vi "mean.vi"(11 "Array":i16[][](array[numeric])) -> (3 "mean":dbl)   [LabVIEW 2015]
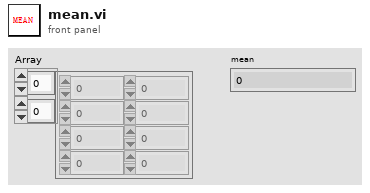
[diagram p1: front panel]
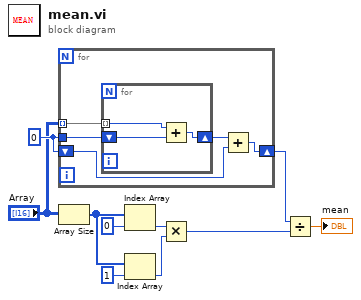
[diagram p0: block diagram]
diagram:
  w5 = i64 0
  n1 = for {
    tunnel: "Array" -> [w15] mode=indexing
    shift-right: [w11] -> w4
    shift-left: w5 -> [w13]
    tunnel: w5 -> [w12]
    n2 = for {
      tunnel: w15 -> [w18] mode=indexing
      shift-right: [w16] -> w14
      shift-left: w12 -> [w17]
      n3 = Add(x=w18, y=w17) -> (x+y=w16:i64)
    }
    n4 = Add(x=w14, y=w13) -> (x+y=w11:i64)
  }
  n5 = Array Size(array="Array") -> (size(s)=w8:i32[])
  n6 = Index Array(array=w8, index=0) -> (element=w7:i32)
  n7 = Index Array(array=w8, index=1) -> (element=w6:i32)
  n8 = Multiply(x=w7, y=w6) -> (x*y=w3:i32)
  n9 = Divide(x=w4, y=w3) -> (x/y=→"mean":dbl)
